vi "D Set Clock-Calender .vi"(4 "Time Stamps(Off:F)":bool, 6 "Time(12:00:00)":string="12:00:00", 7 "Year(1996)":u32=1996 min=1000 max=9999, 8 "error in (no error)":errorcluster, 9 "Day(15)":u32=15 max=31, 10 "Month (January:0)":u16(ring) items=["January", "February", "March", "April", "May", "June", "July", "August", "September", "October", "November", "December"], 11 "VISA resource name":refnum<visa-resource-name>) -> (0 "error out":errorcluster, 3 "VISA resource name out":refnum<visa-resource-name>)   [LabVIEW 2018, in "Agilent 87XX Series.lvlib"]
doc: "This VI sets the time and date on the network analyzer. This vi only works on the 8753D."
uses:
  Agilent 87XX Series.lvlib
panel:
  # "On"
  # "Off"
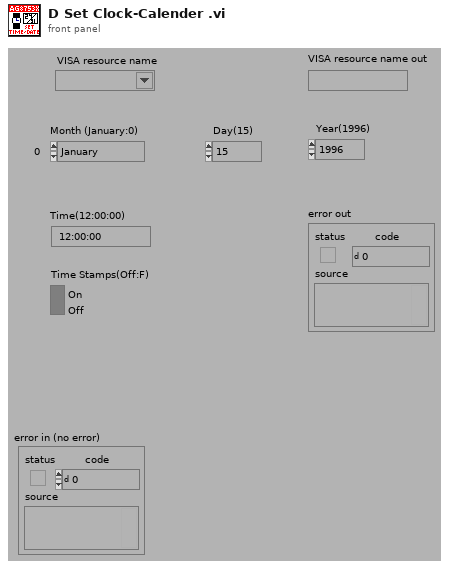
[diagram p1: front panel]
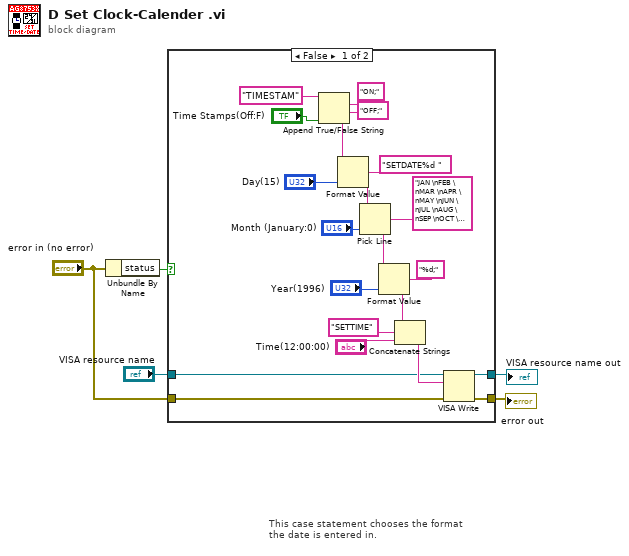
[diagram p0: block diagram]
diagram:
  # "This case statement chooses the format \nthe date is entered in."
  n1 = Unbundle By Name("error in (no error)") -> ("status"=w5:bool)
  n2 = case shown="False" w5 {
    tunnel: [w14 w28] -> w4
    tunnel: [w13 w27] -> w3
    tunnel: "VISA resource name" -> [w12 w28]
    tunnel: "error in (no error)" -> [w11 w27]
    frame False {
      n3 = Append True/False String(1:"Time Stamps(Off:F)", 2:"OFF;", 3:"ON;", 4:"TIMESTAM") -> (0:w10:string)
      n4 = Format Value(string ("")=w10, format string="SETDATE%d ", value (0)="Day(15)") -> (output string=w24:string)
      n5 = Pick Line(string ("")=w24, multi-line string="JAN \nFEB \nMAR \nAPR \nMAY \nJUN \nJUL \nAUG \nSEP \nOCT \nNOV \nDEC ", line index="Month (January:0)") -> (output string=w21:string)
      n6 = Format Value(string ("")=w21, format string="%d;", value (0)="Year(1996)") -> (output string=w18:string)
      n7 = Concatenate Strings(w18, "SETTIME", "Time(12:00:00)") -> (w15:string)
      n8 = VISA Write(VISA resource name=w12, write buffer=w15, error in (no error)=w11) -> (VISA resource name out=w14:refnum<visa-resource-name>, error out=w13:errorcluster)  [unwired: 1 out]
    }
    frame True {
    }
  }
  "VISA resource name out" <- w4
  "error out" <- w3
